vi "test Invalid Event References Leaking.vi"(8 "error in":errorcluster) -> (0 "error out":errorcluster)   [LabVIEW 2020, in "serenial.io-ase.test.lvlib"]
uses:
  serenial.io-ase.test.lvlib
  <vilib>/addons/_JKI Toolkits/Caraya/classes/Assert/Assert.lvclass
  serenial.io-ase/ase/ase.lvclass
  <vilib>/addons/_JKI Toolkits/Caraya/classes/Test/Test.lvclass
  <vilib>/addons/_JKI Toolkits/Caraya/classes/Assert/Assert Equal Value_Variant.vi
  serenial.io-ase/ase/Start Call (Exe-Args).vi
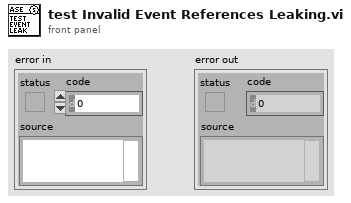
[diagram p1: front panel]
types:
  T1 = typedef "serenial.io-ase.lvlib/ase.lvclass/Event References.ctl" = cluster{"Standard Output":refnum<user-event>, "Standard Error":refnum<user-event>, "Did Exit":refnum<user-event>}
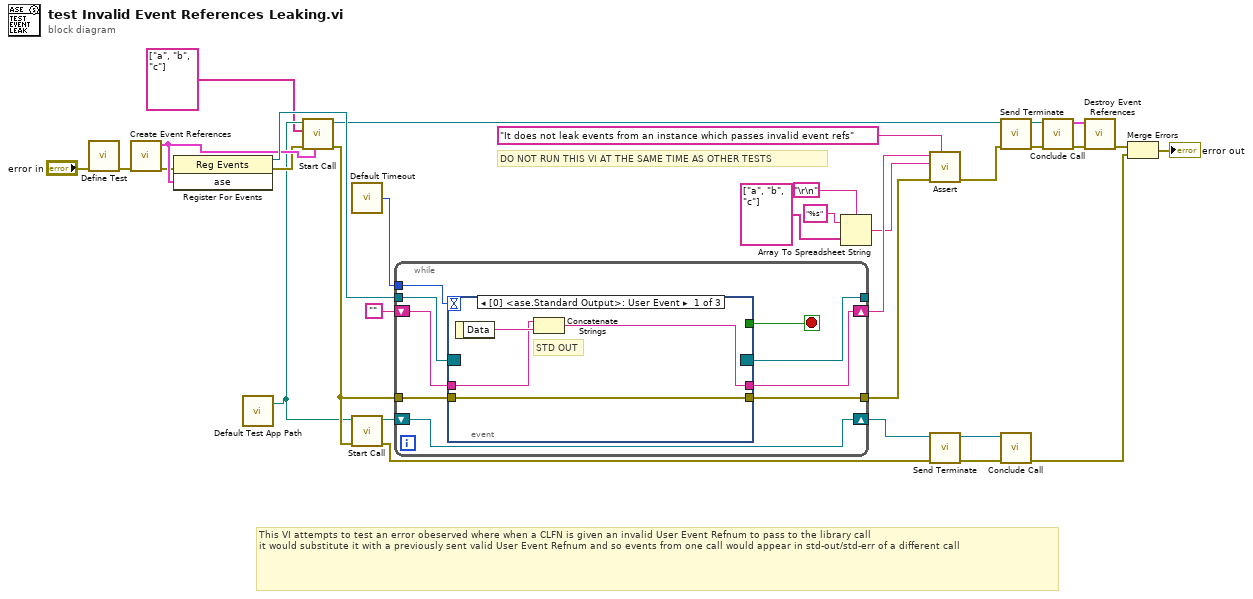
[diagram p0: block diagram]
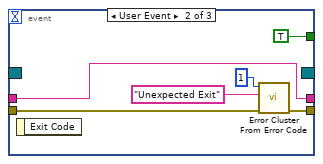
[diagram p2: hidden frame]
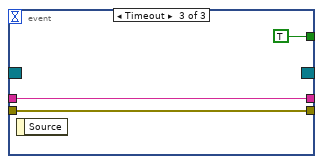
[diagram p3: hidden frame]
diagram:
  # "This VI attempts to test an error obeserved where when a CLFN is given an invalid User Event Refnum to pass to the library call\nit would substitute it with a previously sent valid User Event Refnum and so events from one call would appear in std-out/std-err of a different call"
  # "DO NOT RUN THIS VI AT THE SAME TIME AS OTHER TESTS"
  n1 = call <vilib>:"Define Test.vi"("error in (no error)"="error in") -> ("error out"=w26:errorcluster)  [unwired: 10 in]
  n2 = call "Create Event References.vi"("error in"=w26) -> ("error out"=w24:errorcluster, "ase"=w27:T1)  [unwired: 9 in]
  n3 = register-events(error in=w24, w27) -> (reference out=w29:refnum<event-registration>, error out=w25:errorcluster)  [unwired: 1 in]
  n4 = call "Default Test App Path.vi"() -> ("Exe Path With Extention"=w2:path)  [unwired: 2 in, 1 out]
  n5 = call-poly "Start Call.vi"("Event References"=w27, "error in"=w25, "Arguments"=string[] ["a", "b", "c"], "Executable Path"=w2) -> ("error out"=w14:errorcluster, "New ASE Handle"=w16:refnum<class "ase.lvclass">)  [unwired: 6 in]
  n6 = call "Default Timeout.vi"() -> ("Default Timeout"=w30:i32)
  n7 = call-poly "Start Call.vi"("error in"=w14, "Executable Path"=w2) -> ("error out"=w13:errorcluster, "New ASE Handle"=w11:refnum<class "ase.lvclass">)  [unwired: 8 in]
  n8 = while {
    tunnel: w29 -> [w40]
    tunnel: [w39] -> _
    shift-right: [w36] -> w20
    shift-left: "" ("Empty String Constant") -> [w37]
    tunnel: w30 -> [w35]
    tunnel: [w41] -> w19
    tunnel: w14 -> [w34]
    shift-right: [w33] -> w12
    shift-left: w11 -> [w33]
    stop <- w38 stop-if-true
    n9 = event shown="[0] <ase.Standard Output>: User Event" {
      selector: w40 -> [_ _ _]
      dyn-events: [_ _ _] -> w39
      timeout: w35 -> [_ _ _]
      tunnel: [w42 w49 w52] -> w41
      tunnel: [_ TRUE TRUE] -> w38
      tunnel: w37 -> [w44 w51 w53]
      tunnel: [w43 w51 w53] -> w36
      tunnel: w34 -> [w42 w46 w52]
      event User Event {
        # "STD OUT"
        n10 = event-data() -> ("Data"=w45:string)  [unwired: 1 in]
        n11 = Concatenate Strings(w44, w45) -> (w43:string)
      }
      event User Event {
        n12 = event-data() -> ()  [unwired: 1 in, 1 out]
        n13 = call <vilib>:"Error Cluster From Error Code.vi"("error in (no error)"=w46, "error message (\"\")"="Unexpected Exit" ("error message (\"\")"), "error code (0)"=1) -> ("error out"=w49:errorcluster)  [unwired: 6 in]
      }
      event Timeout {
        n14 = event-data() -> ()  [unwired: 1 in, 1 out]
      }
    }
  }
  n15 = Array To Spreadsheet String(delimiter (Tab)="\r\n", array=string[] ["a", "b", "c"] ("Arguments"), 3:"%s" ("format string")) -> (spreadsheet string=w3:string)
  n16 = call-poly <vilib>:"Assert.vi"("Label"="It does not leak events from an instance which passes invalid event refs", "error in (no error)"=w19, "Y"=w3, "X"=w20) -> ("error out"=w23:errorcluster)  [unwired: 7 in]
  n17 = call "Send Terminate.vi"("error in"=w13, "ASE Handle"=w12) -> ("error out"=w9:errorcluster, "ASE Handle Duplicate"=w10:refnum<class "ase.lvclass">)  [unwired: 7 in, 1 out]
  n18 = call "Send Terminate.vi"("error in"=w23, "ASE Handle"=w16) -> ("error out"=w17:errorcluster, "ASE Handle Duplicate"=w15:refnum<class "ase.lvclass">)  [unwired: 7 in, 1 out]
  n19 = call "Conclude Call.vi"("error in"=w9, "ASE Handle"=w10) -> ("error out"=w7:errorcluster)  [unwired: 7 in, 2 out]
  n20 = call "Conclude Call.vi"("error in"=w17, "ASE Handle"=w15) -> ("error out"=w22:errorcluster, "Event References"=w18:T1)  [unwired: 7 in, 1 out]
  n21 = call "Destroy Event References.vi"("error in"=w22, "Event References"=w18) -> ("error out"=w21:errorcluster)  [unwired: 9 in]
  n22 = Merge Errors(w21, w7) -> (→"error out":errorcluster)
